vi "createCommandListForCommandCase.vi"(7 "timeout (optional)":i32, 9 "immediate Check (only once)":bool=TRUE, 10 "setvalue":string, 11 "command":string) -> (3 "new commands":string)   [LabVIEW 2011]
panel:
  # "must be default 0!!!"
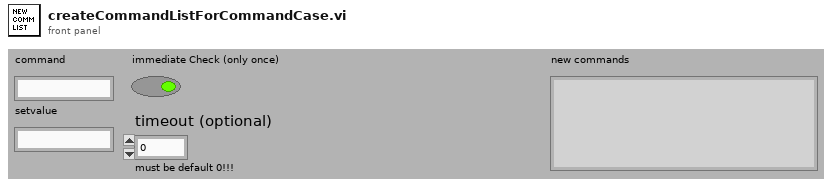
[diagram p1: front panel]
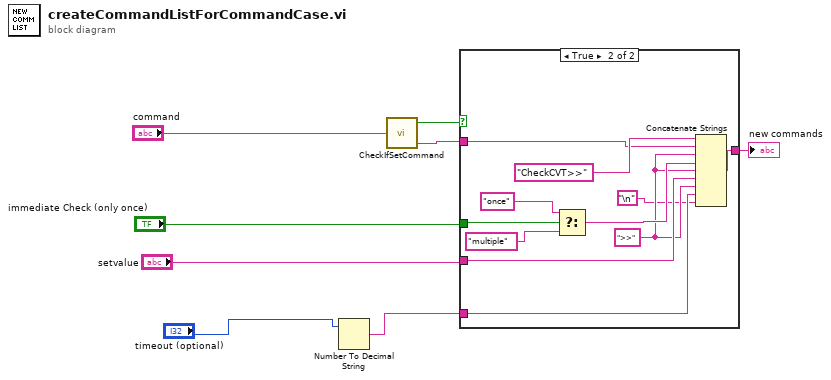
[diagram p0: block diagram]
diagram:
  n1 = Number To Decimal String(number="timeout (optional)") -> (decimal integer string=w1:string)  [unwired: 1 in]
  n2 = call "CheckIfSetCommand.vi"("Command"="command") -> ("setCommand?"=w7:bool, "variable"=w6:string)  [unwired: 1 out]
  n3 = case shown="True" w7 {
    tunnel: w6 -> [_ w15]
    tunnel: "immediate Check (only once)" -> [_ w18]
    tunnel: "setvalue" -> [_ w13]
    tunnel: [_ w12] -> w3
    tunnel: w1 -> [_ w10]
    frame False {
    }
    frame True {
      w11 = ">>" ("string")
      n4 = Select(t="once" ("string"), s=w18, f="multiple" ("string")) -> (s? t:f=w14:string)
      n5 = Concatenate Strings("CheckCVT>>", w15, w11, w14, w11, w13, w11, w10, "\n") -> (w12:string)
    }
  }
  "new commands" <- w3
